vi "5-4 funzioni stringhe.vi"(0 "string 1":string="Range = ", 1 "string":string="conta i caratteri", 2 "multi-string":string="Volt DC\nVolt AC \nResit. (ohms)", 3 "line index":i32, 5 "num":string="10", 7 "string 2":string=" volt", 9 "string in":string="Range = 10 volt", 11 "length (rest)":i32, 12 "sel":bool, 13 "string":string="Selected ") -> (4 "size":i32, 6 "string out":string, 8 "sting out":string, 10 "sting out":string, 15 "out string":string)   [LabVIEW 2012]
doc: "© Copyright M. Ferrari 2002\nString Functions"
panel:
  in  "sel 2":bool
  in  "string 3":string="Beep "
  out "out string 2":string
  in  "F string 2":string="OFF"
  in  "T string 2":string="ON"
  in  "string":string="Beep "
  in  "F string":string="OFF"
  in  "T string":string="ON"
  # "Stringa concatenata"
  # "String subset (valore numerico)"
  # "Selected ......"
  # "Beep ....."
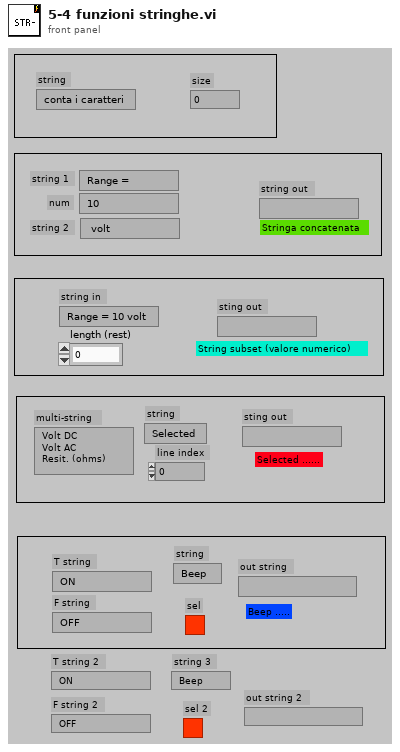
[diagram p1: front panel]
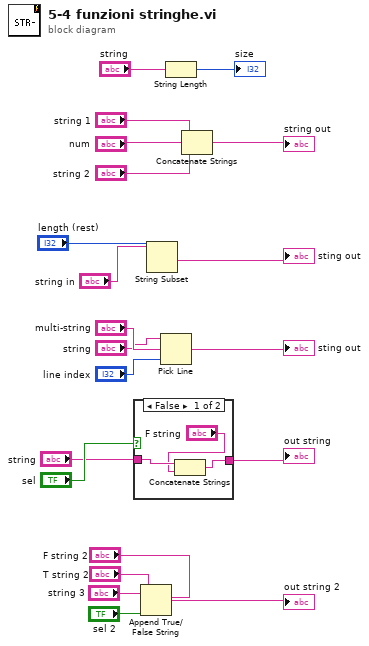
[diagram p0: block diagram]
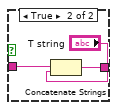
[diagram p2: hidden frame]
diagram:
  n1 = case shown="False" "sel" {
    tunnel: "string" -> [w23 w27]
    tunnel: [w24 w25] -> w8
    frame False {
      n2 = Concatenate Strings(w23, "F string") -> (w24:string)
    }
    frame True {
      n3 = Concatenate Strings(w27, "T string") -> (w25:string)
    }
  }
  "out string" <- w8
  n4 = Append True/False String(1:"sel 2", 2:"F string 2", 3:"T string 2", 4:"string 3") -> (0:→"out string 2":string)
  n5 = String Subset(string="string in", length (rest)="length (rest)") -> (substring=→"sting out":string)  [unwired: 1 in]
  n6 = Pick Line(string ("")="string", multi-line string="multi-string", line index="line index") -> (output string=→"sting out":string)
  n7 = String Length(string="string") -> (length=→"size":i32)
  n8 = Concatenate Strings("string 1", "num", "string 2") -> (→"string out":string)
